vi "Get single frame.vi"(8 "Error In":errorcluster, 11 "Signal Channel":enum16{"Red", "Green"}(ring)) -> (0 "Error Out":errorcluster, 3 "Image":T1(plugin-control))   [LabVIEW 2020]
uses:
  Typedefs/Top level VI states.ctl
  Global Variables/gl_Images.vi
  <vilib>/vision/NI_Vision_Development_Module.lvlib
panel:
  in  "Delay":u32=1000
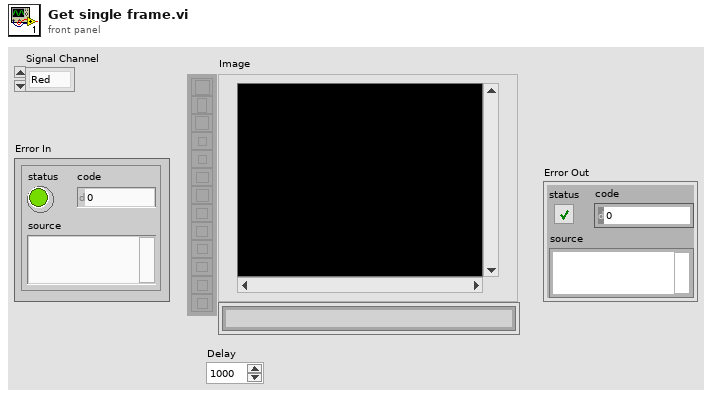
[diagram p1: front panel]
types:
  T1 = typedef "IMAQ Image.ctl" = refnum<image>
  T2 = typedef "Top level VI states.ctl" = enum16{"None", "Initialise UI", "<STACK PROTOCOL STATES>", "AOL Zstack-START", "AOL Zstack-STOP", "Motor Zstack-START", "Motor Zstack-STOP", "Parameter Sweep-START", "Parameter Sweep-STOP", "<ACQUISITION PROTOCOL STATES> ", "Functional Acquisition-START", "Functional Acquisition-STOP", "Single Plane Acquisition-START", "Single Plane Acquisition-STOP", "Volume Acquisition-START", "Volume Acquisition-STOP", "<LIVE IMAGING PROTOCOL STATES>", "Live Imaging-START", "Live Imaging-STOP", "Live Plane Imaging-START", "Live Plane Imaging-STOP", "Live Volume Imaging-START", "Live Volume Imaging-STOP", "<MOVEMENT CORRECTION PROTOCOL STATES>", "EXIT"}
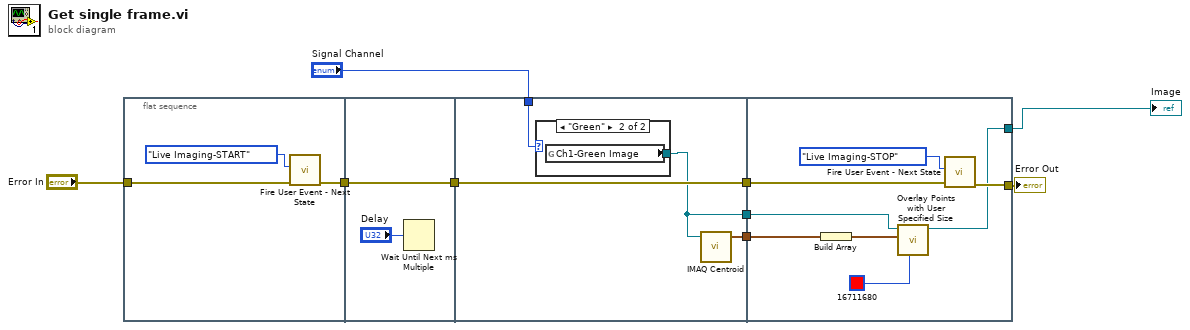
[diagram p0: block diagram]
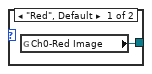
[diagram p2: hidden frame]
diagram:
  n1 = flat-sequence {
    tunnel: "Error In" -> [w11]
    tunnel: [w10] -> w2
    tunnel: w2 -> [w14]
    tunnel: [w14] -> w1
    tunnel: w1 -> [w18]
    tunnel: [w18] -> w8
    tunnel: "Signal Channel" -> [w17]
    tunnel: [w16] -> w4
    tunnel: [w15] -> w3
    tunnel: w8 -> [w27]
    tunnel: [w26] -> w7
    tunnel: [w21] -> w5
    tunnel: w4 -> [w24]
    tunnel: w3 -> [w25]
    frame #0 {
      n2 = call "Fire User Event - Next State.vi"("Error In"=w11, "\"UI Handler loop\" case to execute"=Top_level_VI_states."Live Imaging-START" ("\"UI Handler loop\" case to execute")) -> ("Error Out"=w10:errorcluster)  [unwired: 9 in]
    }
    frame #1 {
      n3 = Wait Until Next ms Multiple(millisecond multiple="Delay") -> ()  [unwired: 1 out]
    }
    frame #2 {
      n4 = case shown="\"Green\"" w17 {
        tunnel: [w19 w20] -> w15
        frame "Red", Default {
          n5 = global read "gl_Images.vi" "Ch0-Red Image"() -> (w19:T1)
        }
        frame "Green" {
          n6 = global read "gl_Images.vi" "Ch1-Green Image"() -> (w20:T1)
        }
      }
      n7 = call "IMAQ Centroid"("Image"=w15) -> ("Centroid"=w16:cluster{"X Centroid":sgl, "Y Centroid":sgl})  [unwired: 3 in, 1 out]
    }
    frame #3 {
      n8 = Build Array(w24) -> (w23:cluster{"X Centroid":sgl, "Y Centroid":sgl}[])
      n9 = call "Overlay Points with User Specified Size.vi"("Color"=u32 16711680, "Points"=w23, "Image In"=w25) -> ("Image Out"=w21:T1)  [unwired: 7 in, 1 out]
      n10 = call "Fire User Event - Next State.vi"("Error In"=w27, "\"UI Handler loop\" case to execute"=Top_level_VI_states."Live Imaging-STOP" ("\"UI Handler loop\" case to execute")) -> ("Error Out"=w26:errorcluster)  [unwired: 9 in]
    }
  }
  "Error Out" <- w7
  "Image" <- w5
